vi "Set Counter Input.vi"(8 "error in (no error)":errorcluster, 9 "Input (def: 10 MHz)":enum16{"10 MHz", "INPUT 1", "INPUT 2", "TRIG"}(ring), 10 "Counter (def: A)":T1, 11 "VISA resource name":refnum<visa-resource-name>) -> (0 "error out":errorcluster, 3 "VISA resource name out":refnum<visa-resource-name>)   [LabVIEW 2015, in "SR400.lvlib"]
uses:
  SR400.lvlib
  Typedefs/Counter.ctl
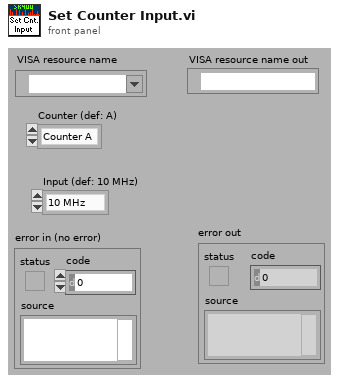
[diagram p1: front panel]
types:
  T1 = typedef "SR400.lvlib/Counter.ctl" = enum16{"Counter A", "Counter B", "Counter T"}
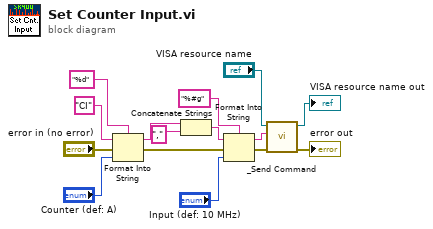
[diagram p0: block diagram]
diagram:
  n1 = Format Into String(format string="%d", initial string="CI" ("command"), error in="error in (no error)", "Counter (def: A)") -> (resulting string=w8:string, error out=w7:errorcluster)
  n2 = Concatenate Strings(w8, "," ("command")) -> (w13:string)
  n3 = Format Into String(format string="%#g", initial string=w13, error in=w7, "Input (def: 10 MHz)") -> (resulting string=w4:string, error out=w3:errorcluster)
  n4 = call "_Send Command.vi"("error in (no error)"=w3, "Command"=w4, "VISA resource name"="VISA resource name") -> ("error out"=→"error out":errorcluster, "VISA resource name out"=→"VISA resource name out":refnum<visa-resource-name>)  [unwired: 1 in, 6 out]
